vi "Dateischreiben_Echtes_Signal_MessWerte.vi"() -> ()   [LabVIEW 2016]
panel:
  out "PT":dbl
  out "Te":dbl
  in  "Messfrequenz":dbl=10.0
  in  "Spalten":string[](array[string])=["y-wert\n", "", "", ""]
  in  "Header":string[](array[string])=["Messlabor\n", "trajan_ursiwn", "21092023", "HTBLA Kaindorf"]
  out "Signalverlauf":dynamicdata(graph)
  in  "Eingangs-String":string="%f\\t%f\\t%f\\t%f\\t%f\\n"
  in  "Pfad":path=path "C:/Users/Messlabor_Kustos/Desktop/Schueler/4BHME/28.09.2023/DatenTabelleMessWerte.xls"
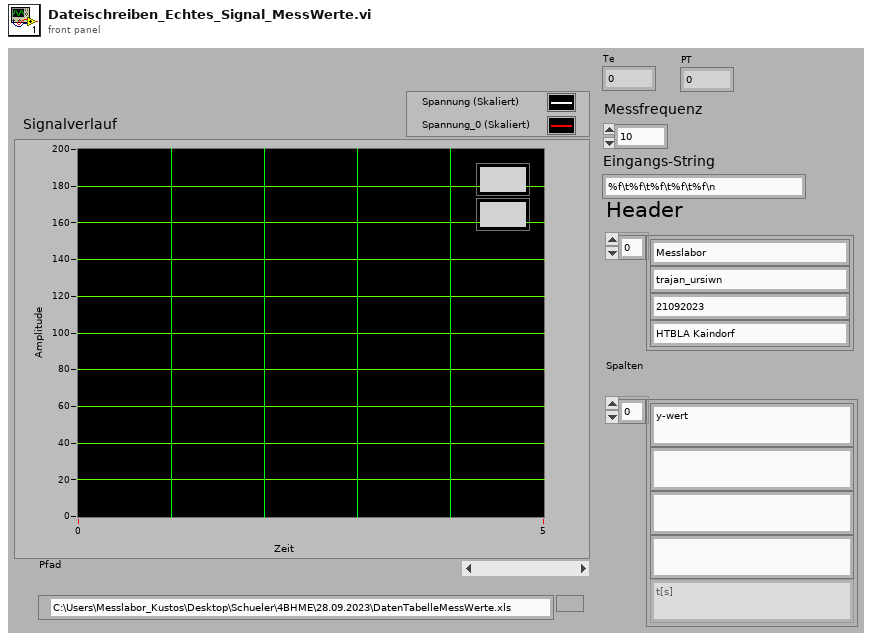
[diagram p1: front panel]
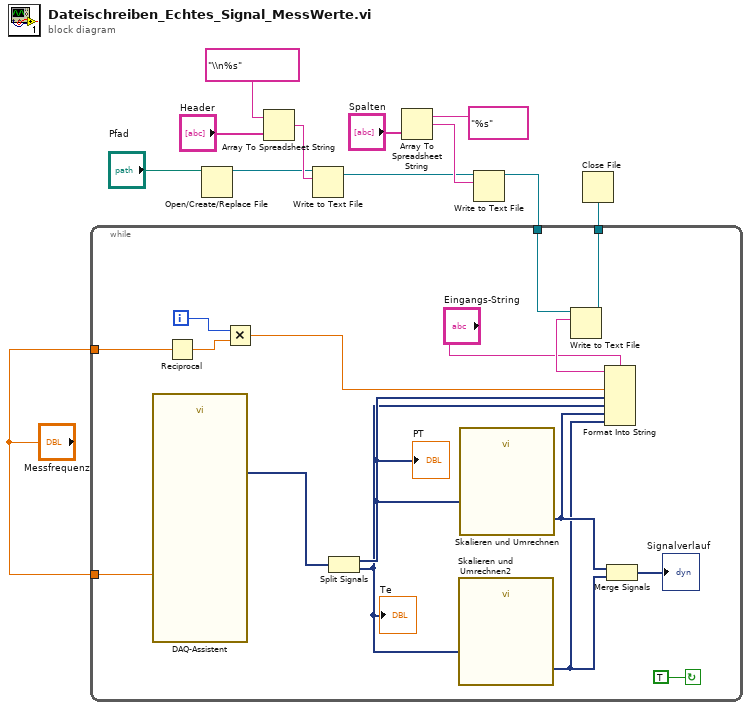
[diagram p0: block diagram]
diagram:
  n1 = Open/Create/Replace File(file path (use dialog)="Pfad") -> (refnum out=w4:refnum<file>)  [unwired: 5 in, 2 out]
  n2 = Array To Spreadsheet String(array="Header", 3:"\\n%s" ("Format-String")) -> (spreadsheet string=w6:string)  [unwired: 1 in]
  n3 = Write to Text File(file (use dialog)=w4, text=w6) -> (refnum out=w2:refnum<file>)  [unwired: 2 in, 2 out]
  n4 = Array To Spreadsheet String(array="Spalten", 3:"%s" ("Format-String")) -> (spreadsheet string=w5:string)  [unwired: 1 in]
  n5 = Write to Text File(file (use dialog)=w2, text=w5) -> (refnum out=w3:refnum<file>)  [unwired: 2 in, 2 out]
  n6 = while {
    tunnel: [w28] -> w12
    tunnel: w3 -> [w24]
    tunnel: "Messfrequenz" -> [w23]
    tunnel: "Messfrequenz" -> [w14]
    i -> [w21]
    stop <- TRUE continue-if-true
    n7 = call "DAQ-Assistent"("Rate"=w14) -> ("data"=w13:dynamicdata)  [unwired: 15 in, 3 out]
    n8 = Reciprocal(x=w23) -> (1/x=w22:dbl)
    n9 = Multiply(x=w21, y=w22) -> (x*y=w20:dbl)
    n10 = Split Signals(w13) -> (w18:dynamicdata, w17:dynamicdata)  [unwired: 2 in]
    "Te" <- w17
    "PT" <- w18
    n11 = call "Skalieren und Umrechnen2"("Signals"=w17) -> ("Scaled Signals"=w15:dynamicdata)  [unwired: 9 in, 1 out]
    n12 = call "Skalieren und Umrechnen"("Signals"=w18) -> ("Scaled Signals"=w16:dynamicdata)  [unwired: 9 in, 1 out]
    n13 = Format Into String(format string="Eingangs-String", w20, w18, w17, w16, w15) -> (resulting string=w27:string)  [unwired: 2 in, 1 out]
    n14 = Write to Text File(file (use dialog)=w24, text=w27) -> (refnum out=w28:refnum<file>)  [unwired: 2 in, 2 out]
    n15 = Merge Signals(w16, w15) -> (→"Signalverlauf":dynamicdata)
  }
  n16 = Close File(refnum=w12) -> ()  [unwired: 1 in, 2 out]
